vi "TCPSerialInterfaceData.vi"(0 "整体更新":T1(c390), 1 "信息":T3, 10 "客服接口枚举":enum16{"ini", "增", "删", "查", "改", "腾笼换鸟"}(ring)) -> (14 "服务表":T1(c390), 17 "查找结果":T2)   [LabVIEW 2019]
uses:
  02 Mode/TCPServerMode/TCPServerClass.lvclass
  <vilib>/Utility/miscctls.llb/LVMapReplaceAction.ctl
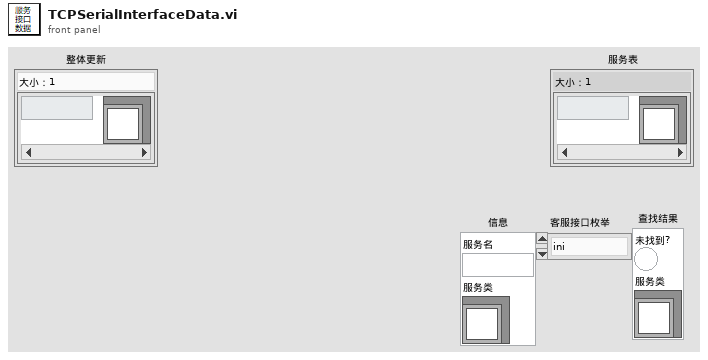
[diagram p1: front panel]
types:
  T1 = map{string, refnum<class "TCPServerClass.lvclass">}
  T2 = cluster{"未找到?":bool, "服务类":refnum<class "TCPServerClass.lvclass">}
  T3 = cluster{"服务名":string, "服务类":refnum<class "TCPServerClass.lvclass">}
  T4 = typedef "LVMapReplaceAction.ctl" = enum32{"Modify Entry only if found", "Add or Modify Entry", "Delete Entry"}
  T5 = cluster{"key not found?":bool, "TCPServerClass.lvclass":refnum<class "TCPServerClass.lvclass">}
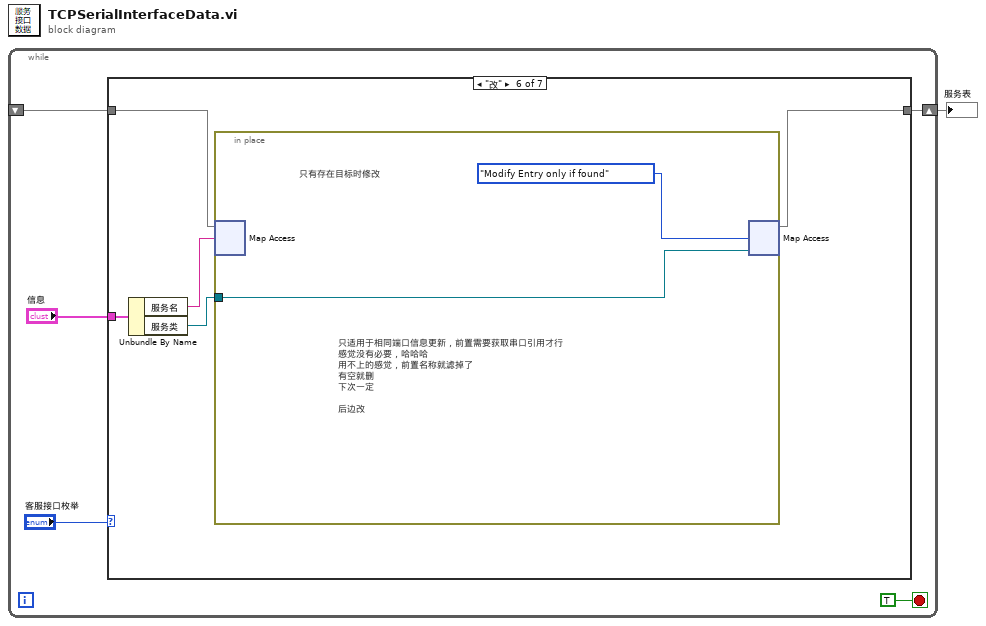
[diagram p0: block diagram]
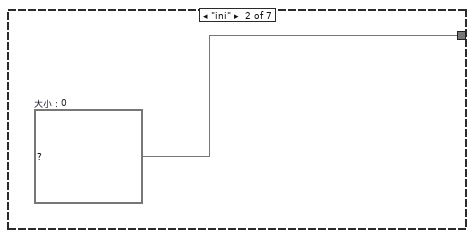
[diagram p3: hidden frame]
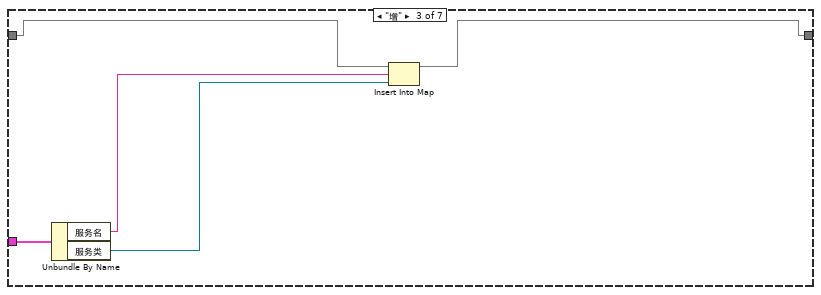
[diagram p4: hidden frame]
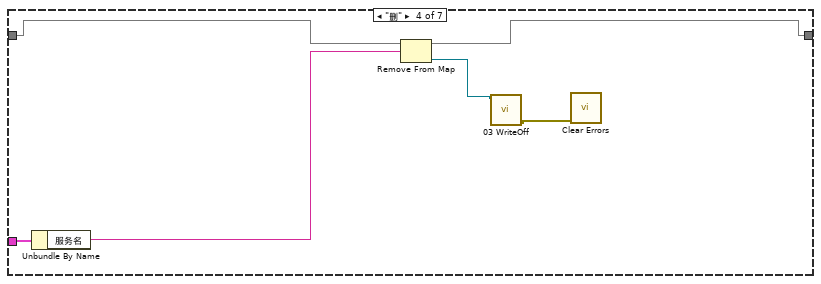
[diagram p5: hidden frame]
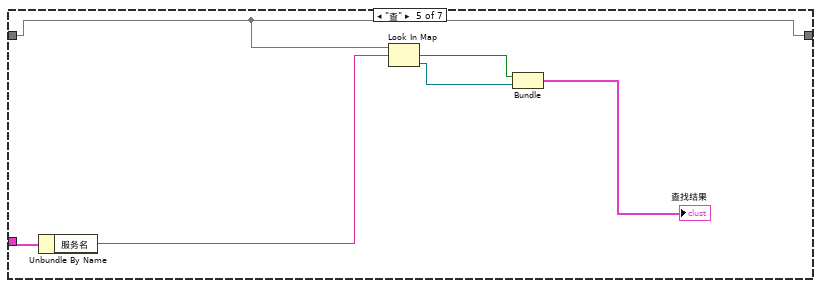
[diagram p6: hidden frame]
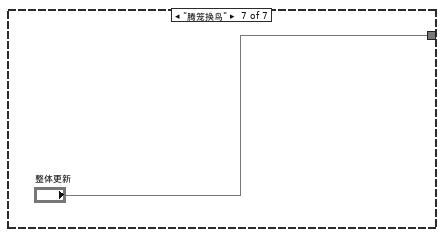
[diagram p7: hidden frame]
diagram:
  n1 = while {
    shift-right: [w3] -> w1
    shift-left: _ -> [w2]
    stop <- TRUE stop-if-true
    n2 = case shown="\"改\"" "客服接口枚举" {
      tunnel: "信息" -> [_ _ w13 w19 w25 w30 _]
      tunnel: [w7 w8 w9 w16 w20 w26 "整体更新"] -> w3
      tunnel: w2 -> [w7 _ w10 w17 w20 w27 _]
      frame Default {
      }
      frame "ini" {
        w8 = T1 {}  # 大小：0
      }
      frame "增" {
        n3 = Unbundle By Name(w13) -> ("服务名"=w12:string, "服务类"=w11:refnum<class "TCPServerClass.lvclass">)
        n4 = Insert Into Map(map in=w10, key=w12, value=w11) -> (map out=w9:T1)  [unwired: 2 out]
      }
      frame "删" {
        n5 = Unbundle By Name(w19) -> ("服务名"=w18:string)
        n6 = Remove From Map(10:w18, 11:w17) -> (1:w15:refnum<class "TCPServerClass.lvclass">, 3:w16:T1)  [unwired: 1 out]
        n7 = call-dynamic "03 WriteOff.vi"("TCPServerClass 输入"=w15) -> ("error out"=w14:errorcluster)  [unwired: 9 in, 1 out]
        n8 = call <vilib>:"Clear Errors.vi"("error in (no error)"=w14) -> ()  [unwired: 5 in, 2 out]
      }
      frame "查" {
        n9 = Unbundle By Name(w25) -> ("服务名"=w24:string)
        n10 = Look In Map(map=w20, key=w24) -> (key not found?=w23:bool, value=w22:refnum<class "TCPServerClass.lvclass">)  [unwired: 1 in]
        n11 = Bundle("key not found?"=w23, "TCPServerClass.lvclass"=w22) -> (→"查找结果":T5)  [unwired: 1 in]
      }
      frame "改" {
        n12 = Unbundle By Name(w30) -> ("服务名"=w29:string, "服务类"=w28:refnum<class "TCPServerClass.lvclass">)
        n13 = in-place {
          in-place-border: w28 -> [w31]
          # "只适用于相同端口信息更新，前置需要获取串口引用才行\n感觉没有必要，哈哈哈\n用不上的感觉，前置名称就滤掉了\n有空就删\n下次一定\n\n后边改"
          # "只有存在目标时修改"
          n14 = in-place-map #1(w27, w29) -> ()  [unwired: 1 in, 2 out]
          n15 = in-place-map #1(w31, LVMapReplaceAction."Modify Entry only if found" ("操作")) -> (w26:T1)  [unwired: 2 out]
        }
      }
      frame "腾笼换鸟" {
      }
    }
  }
  "服务表" <- w1
